vi "Device VI 2.0.vi"() -> ()   [LabVIEW 2017]
uses:
  <vilib>/Utility/error.llb/DialogType.ctl
  <vilib>/DAQmx/read.llb/DAQmx Read (Analog 1D Wfm NChan NSamp).vi
  <vilib>/Analysis/5stat.llb/RMS (DBL).vi
  <vilib>/DAQmx/write.llb/DAQmx Write (Digital 1D U8 1Chan NSamp).vi
  <vilib>/DAQmx/create/channels.llb/DAQmx Create Channel (AI-Force-Bridge-Two-Point-Linear).vi
  <vilib>/DAQmx/configure/timing.llb/DAQmx Timing (Sample Clock).vi
  <vilib>/DAQmx/configure/trigger.llb/DAQmx Start Trigger (Digital Edge).vi
  <vilib>/DAQmx/miscellaneous.llb/DAQmx Fill In Error Info.vi
  <vilib>/DAQmx/create/channels.llb/DAQmx Create Channel (DO-Digital Output).vi
  <vilib>/Waveform/WDTFileIO.llb/Export Waveforms To Spreadsheet File (1D).vi
  <resource>/objmgr/daqmx.rc
  <vilib>/Analysis/NI_AALPro.lvlib
panel:
  in  "stop":bool
  in  "Output Array":u32[](array[numeric])=[1, 2, 4, 8, 16, 32, 64, 128]
  in  "Number of Samples":i32=1000
  in  "Sample Rate 2":dbl=1000.0
  in  "Sample Clock Source":tag="PFI0"
  in  "Line(s)":tag="Dev1/port0/line0:7"
  out "rms value":dbl format="%0.2f"
  out "x > y?":bool
  in  "scaling information":T1={"first electrical value"=0.0, "second electrical value"=1.0, "electrical units"=15897, "first physical value"=0.0, "second physical value"=7.39, "physical units"=15876} {"physical units" items=["Newtons"=15875, "Pounds"=15876, "kgf"=15877]; "electrical units" items=["Volts/Volt"=15896, "mVolts/Volt"=15897]}
  in  "Pause":bool
  in  "Start":bool
  in  "Spreadsheet Location":path=path "C:/Users/Julio/Desktop/Device Data/Test.xlsx" caption="Filename"
  in  "Maximum Force":dbl=25.0
  in  "Minimum Force":dbl=-25.0
  in  "Units (Force)":i32(ring)=15876 items=["Newtons"=15875, "Pounds"=15876, "kgf"=15877, "From Custom Scale"=10065]
  in  "Trigger Type":T2(tab)
  in  "Digital Start Trigger Edge":i32(ring)=10280 caption="Edge" items=["Rising"=10280, "Falling"=10171]
  in  "Digital Start Trigger Source":tag="/cDAQ1Mod3/PFI0" caption="Source"
  in  "Digital Pause Trigger Pause When":i32(ring)=10192 caption="Pause When" items=["High"=10192, "Low"=10214]
  in  "Digital Pause Trigger Source":tag="/Dev1/PFI0" caption="Source"
  in  "Bridge Information":T3={"Bridge Configuration"=10182, "Excitation Source"=10200, "Excitation Value"=10.0, "Nominal Resistance"=350.0} {"Excitation Source" items=["Internal"=10200, "External"=10167, "None"=10230]; "Bridge Configuration" items=["Full Bridge"=10182, "Half Bridge"=10187, "Quarter Bridge"=10270, "No Bridge"=10228]}
  in  "Physical Channel":tag="cDAQ1Mod1/ai0:1"
  in  "Sample Rate":dbl=1000.0
  in  "Samples per Loop":i32=500
  out "Waveform Chart":waveform(dbl)[](graph)=[{"t0"=timestamp(3613388787.7661867 s since 1904-01-01), "dt"=0.00062, "Y"=array[500 elements], "attributes"=variant("NI_ChannelName"=variant(string "cDAQ1Mod1/ai0"), "NI_UnitDescription"=variant(string "Pounds"))}, {"t0"=timestamp(3613388787.7661867 s since 1904-01-01), "dt"=0.00062, "Y"=array[500 elements], "attributes"=variant("NI_ChannelName"=variant(string "cDAQ1Mod1/ai1"), "NI_UnitDescription"=variant(string "Pounds"))}]
  # "Settings"
  # "Data"
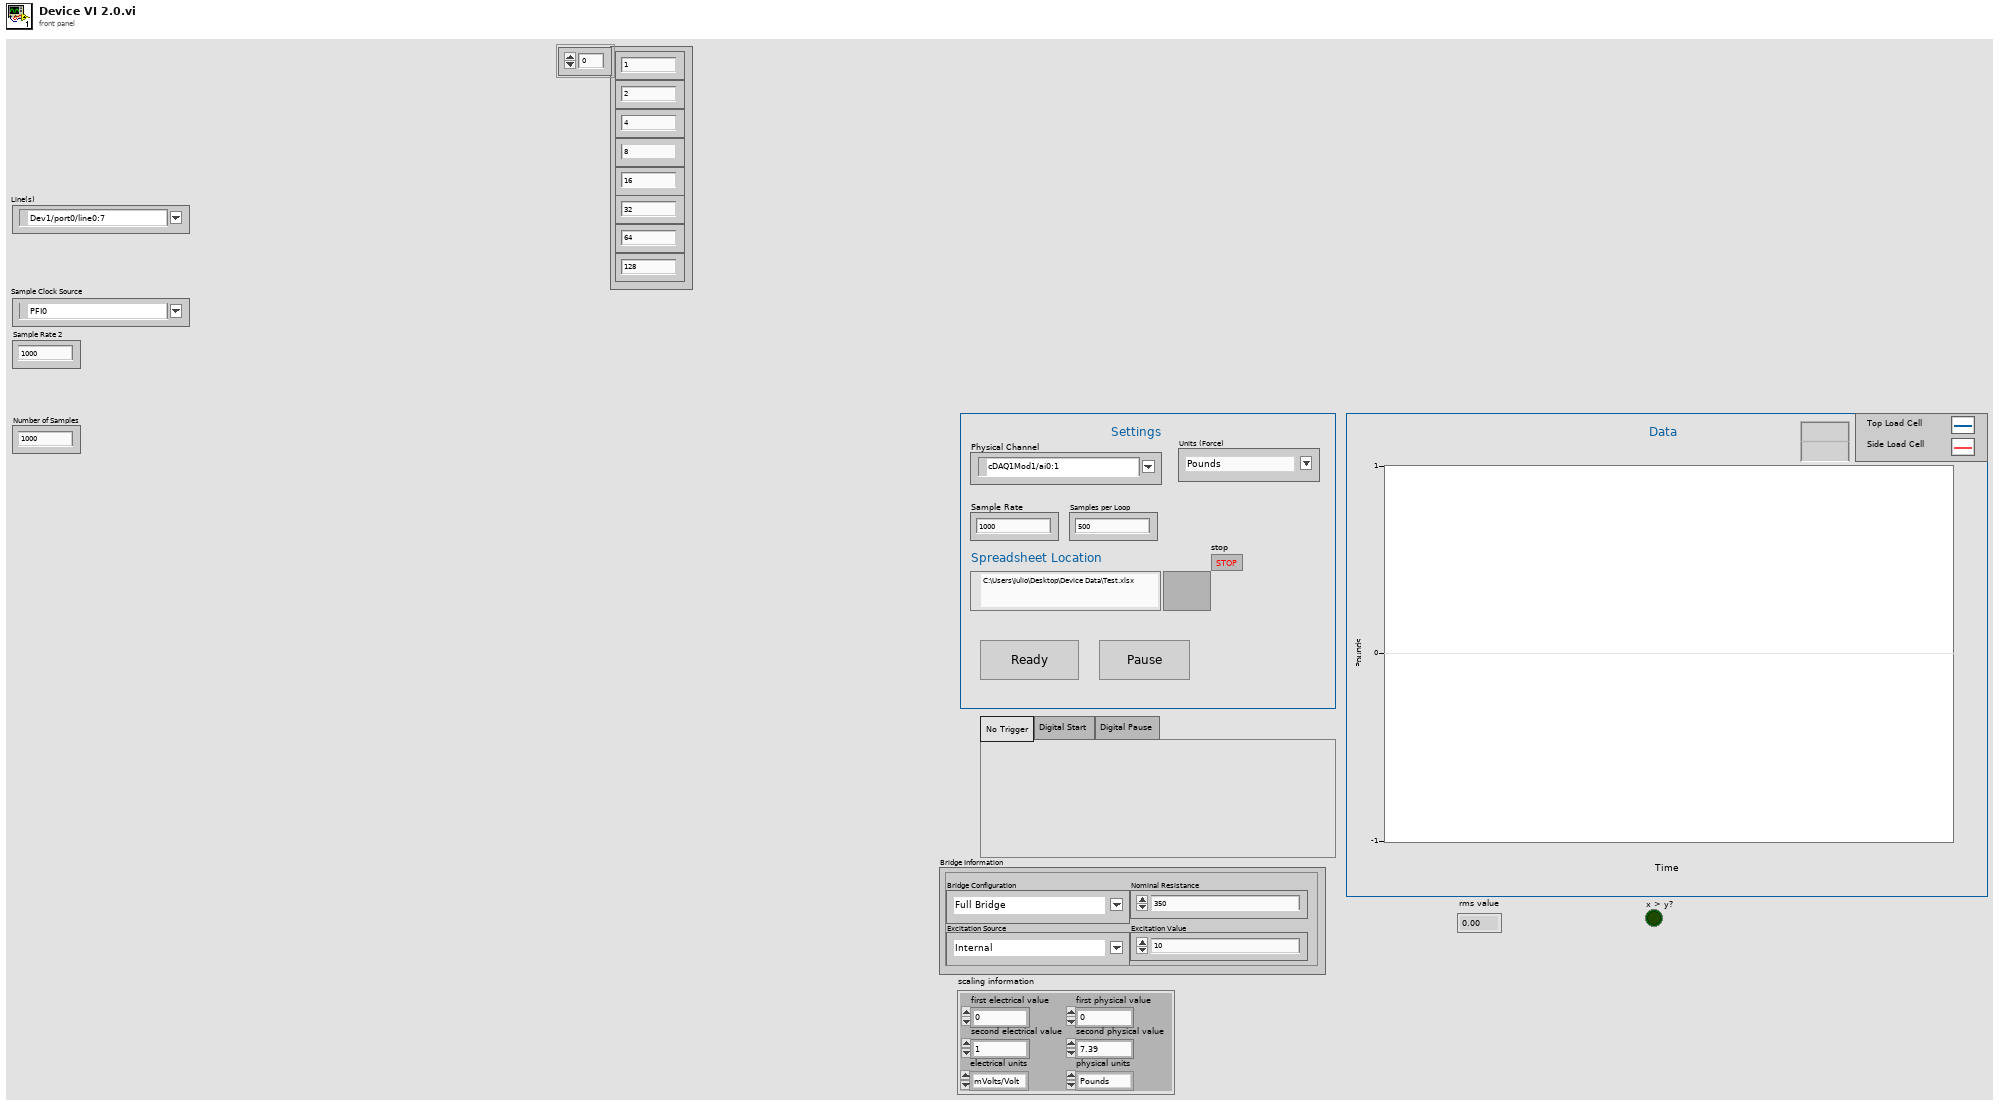
[diagram p1: front panel]
types:
  T1 = cluster{"first electrical value":dbl, "second electrical value":dbl, "electrical units":i32, "first physical value":dbl, "second physical value":dbl, "physical units":i32}
  T2 = enum32{"No Trigger", "Digital Start", "Digital Pause"}
  T3 = cluster{"Bridge Configuration":i32, "Excitation Source":i32, "Excitation Value":dbl, "Nominal Resistance":dbl}
  T4 = typedef "DialogType.ctl" = u16
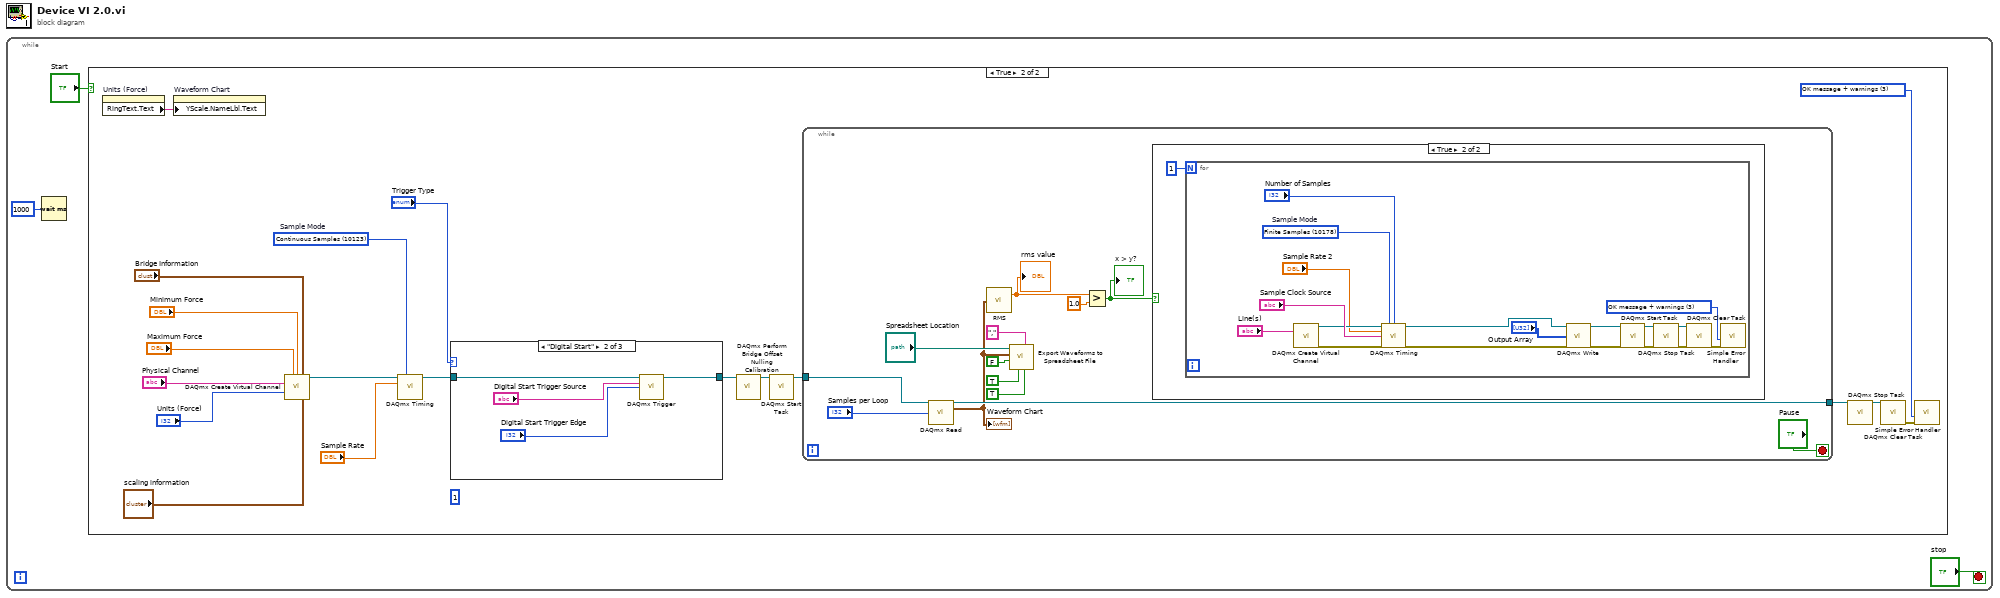
[diagram p0: block diagram]
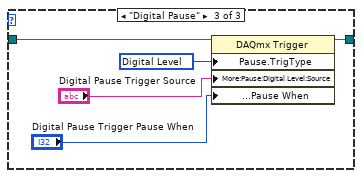
[diagram p4: hidden frame]
diagram:
  n1 = while {
    stop <- "stop" stop-if-true
    n2 = Wait (ms)(milliseconds to wait=u32 1000) -> ()  [unwired: 1 out]
    n3 = case shown="True" "Start" {
      frame False {
      }
      frame True {
        (unwired) 1
        w14 = T4 3 items=["no dialog", "OK message", "continue or stop message", "OK message + warnings", "continue/stop + warnings"] ("type of dialog (OK msg:1)")
        w22 = 10123 items=["Finite Samples"=10178, "Continuous Samples"=10123, "Hardware Timed Single Point"=12522]  # Sample Mode
        n4 = property on="Units (Force)" class="Ring (strict)"() -> ("RingText.Text"=w7:string)  [unwired: 2 in, 2 out]
        n5 = property on="Waveform Chart" class="WFChart (strict)"("YScale.NameLbl.Text"=w7) -> ()  [unwired: 2 in, 2 out]
        n6 = call-poly <vilib>:"DAQmx Create Virtual Channel.vi"("maximum value"="Maximum Force", "minimum value"="Minimum Force", "bridge information"="Bridge Information", "physical channels"="Physical Channel", "units"="Units (Force)", "scaling information"="scaling information") -> ("task out"=w21:refnum<k21>)  [unwired: 8 in, 1 out]
        n7 = call-poly <vilib>:"DAQmx Timing.vi"("task/channels in"=w21, "sample mode"=w22, "rate"="Sample Rate") -> ("task out"=w8:refnum<k21>)  [unwired: 11 in, 1 out]
        n8 = case shown="\"Digital Start\"" "Trigger Type" {
          tunnel: w8 -> [w23 w27 w32]
          tunnel: [w23 w26 w31] -> w12
          frame "No Trigger", Default {
          }
          frame "Digital Start" {
            n9 = call-poly <vilib>:"DAQmx Trigger.vi"("task/channels in"=w27, "source"="Digital Start Trigger Source", "edge"="Digital Start Trigger Edge") -> ("task out"=w26:refnum<k21>)  [unwired: 11 in, 1 out]
          }
          frame "Digital Pause" {
            w30 = 10152 items=["Analog Level"=10101, "Analog Window"=10103, "Digital Level"=10152, "Digital Pattern"=10398, "None"=10230] ("Pause.TrigType")
            n10 = property class="DAQmx Trigger"(reference=w32, "Pause.TrigType"=w30, "More:Pause:Digital Level:Source"="Digital Pause Trigger Source", "More:Pause:Digital Level:Pause When"="Digital Pause Trigger Pause When") -> (reference out=w31:refnum<k21>)  [unwired: 1 in, 1 out]
          }
        }
        n11 = call <vilib>:"DAQmx Perform Bridge Offset Nulling Calibration.vi"("task/channels in"=w12) -> ("task out"=w6:refnum<k21>)  [unwired: 13 in, 1 out]
        n12 = call <vilib>:"DAQmx Start Task.vi"("task/channels in"=w6) -> ("task out"=w20:refnum<k21>)  [unwired: 13 in, 1 out]
        n13 = while {
          tunnel: w20 -> [w45]
          tunnel: [w42] -> w4
          stop <- "Pause" stop-if-true
          n14 = call-poly <vilib>:"DAQmx Read.vi"("task/channels in"=w45, "number of samples per channel"="Samples per Loop") -> ("task out"=w42:refnum<k21>, "data"=w36:waveform(dbl)[])  [unwired: 11 in, 1 out]
          "Waveform Chart" <- w36
          n15 = call-poly <vilib>:"RMS.vi"("X"=w36) -> ("rms value"=w34:dbl)  [unwired: 1 out]
          "rms value" <- w34
          n16 = call-poly <vilib>:"Export Waveforms to Spreadsheet File.vi"("header? (write header:T)"=TRUE, "delimiter (Tab)"=",", "append to file? (new file:F)"=TRUE, "multiple time columns? (single:F)"=FALSE, "waveforms"=w36, "file path (dialog if empty)"="Spreadsheet Location") -> ()  [unwired: 4 in, 2 out]
          n17 = Greater?(x=w34, y=1.0) -> (0:w33:bool)
          "x > y?" <- w33
          n18 = case shown="True" w33 {
            frame False {
            }
            frame True {
              n19 = for {
                N: 1 -> [_]
                w50 = T4 3 items=["no dialog", "OK message", "continue or stop message", "OK message + warnings", "continue/stop + warnings"] ("type of dialog (OK msg:1)")
                w57 = 10178 items=["Finite Samples"=10178, "Continuous Samples"=10123, "Hardware Timed Single Point"=12522]  # Sample Mode
                n20 = call-poly <vilib>:"DAQmx Create Virtual Channel.vi"("lines"="Line(s)") -> ("task out"=w61:refnum<k21>, "error out"=w60:errorcluster)  [unwired: 13 in]
                n21 = call-poly <vilib>:"DAQmx Timing.vi"("task/channels in"=w61, "sample mode"=w57, "samples per channel"="Number of Samples", "rate"="Sample Rate 2", "source"="Sample Clock Source", "error in"=w60) -> ("task out"=w56:refnum<k21>, "error out"=w55:errorcluster)  [unwired: 8 in]
                n22 = call-poly <vilib>:"DAQmx Write.vi"("task/channels in"=w56, "data"="Output Array", "error in"=w55) -> ("task out"=w54:refnum<k21>, "error out"=w53:errorcluster)  [unwired: 10 in, 1 out]
                n23 = call <vilib>:"DAQmx Start Task.vi"("task/channels in"=w54, "error in"=w53) -> ("task out"=w48:refnum<k21>, "error out"=w47:errorcluster)  [unwired: 12 in]
                n24 = call <vilib>:"DAQmx Stop Task.vi"("task/channels in"=w48, "error in"=w47) -> ("task out"=w52:refnum<k21>, "error out"=w51:errorcluster)  [unwired: 12 in]
                n25 = call <vilib>:"DAQmx Clear Task.vi"("task in"=w52, "error in"=w51) -> ("error out"=w64:errorcluster)  [unwired: 13 in]
                n26 = call <vilib>:"Simple Error Handler.vi"("type of dialog (OK msg:1)"=w50, "error in (no error)"=w64) -> ()  [unwired: 3 in, 5 out]
              }
            }
          }
        }
        n27 = call <vilib>:"DAQmx Stop Task.vi"("task/channels in"=w4) -> ("task out"=w15:refnum<k21>)  [unwired: 13 in, 1 out]
        n28 = call <vilib>:"DAQmx Clear Task.vi"("task in"=w15) -> ("error out"=w19:errorcluster)  [unwired: 14 in]
        n29 = call <vilib>:"Simple Error Handler.vi"("type of dialog (OK msg:1)"=w14, "error in (no error)"=w19) -> ()  [unwired: 3 in, 5 out]
      }
    }
  }
